vi "Get Array Elements.vi"(6 "Pass non-arrays":bool, 8 "error in (no error)":errorcluster, 10 "Offset":i32, 11 "JSON":string) -> (0 "error out":errorcluster, 1 "<JSON>":string[](array[string]) caption="<JSON>Elements", 2 "Offset past":i32 caption="Offset past Array")   [LabVIEW 2019, in "JSONtext.lvlib"]
doc: "If a JSON Array, returns all elements of the Array.\n\nIf the input JSON is not an Array, this function will return an error, unless \"Pass non-arrays\" is true, in which case the output will be a one-element array containing the input JSON."
uses:
  JSONtext.lvlib
  Parsing/Parsing State.ctl
  Parsing/Advance past Line Ending.vi
  Parsing/Advance past String.vi
  Parsing/Advance past Number.vi
  Parsing/Advance past Array.vi
  Parsing/Advance past Object.vi
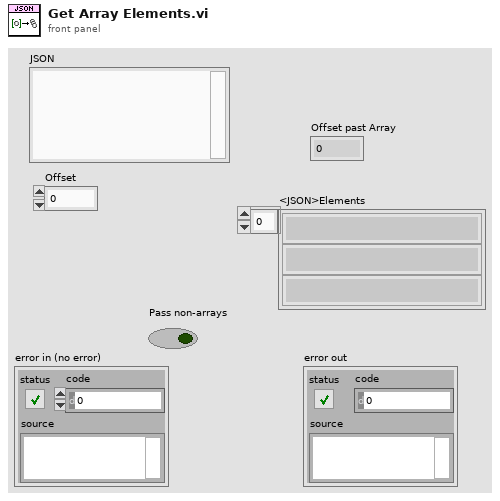
[diagram p1: front panel]
types:
  T1 = typedef "JSONtext.lvlib/Parsing State.ctl" = enum16{"Parser Error", "Object", "Array", "String", "Number/Other", "Leading Whitespace", "Object end", "Array end", "Value end"}
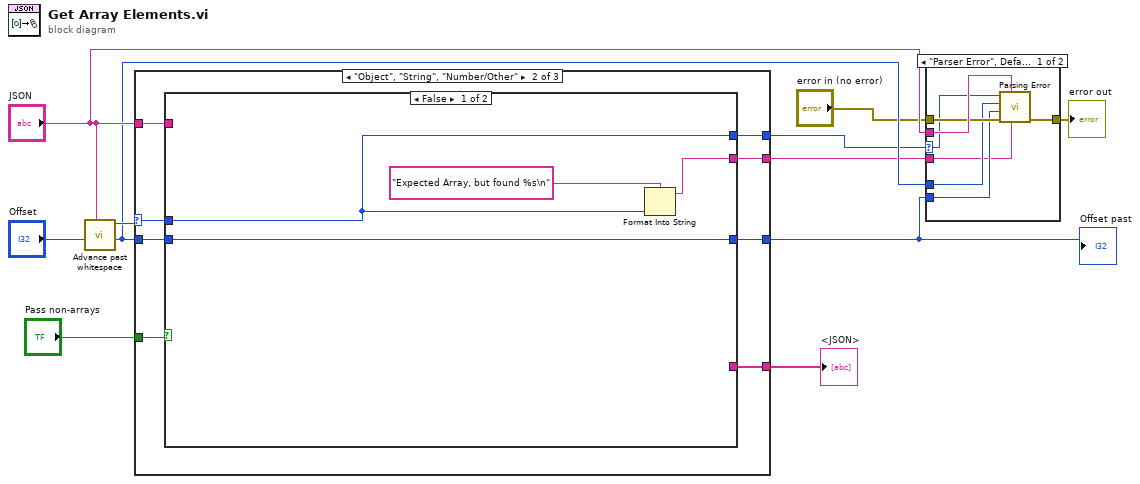
[diagram p0: block diagram]
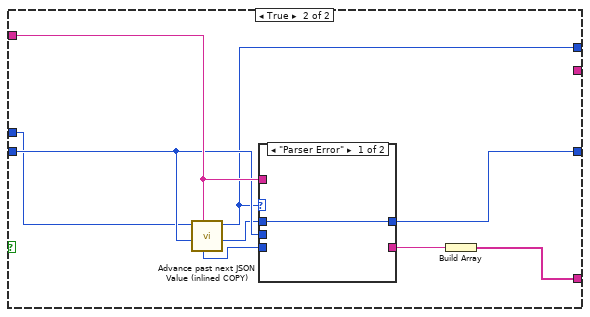
[diagram p4: hidden frame]
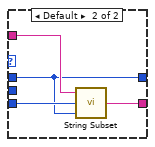
[diagram p5: hidden frame]
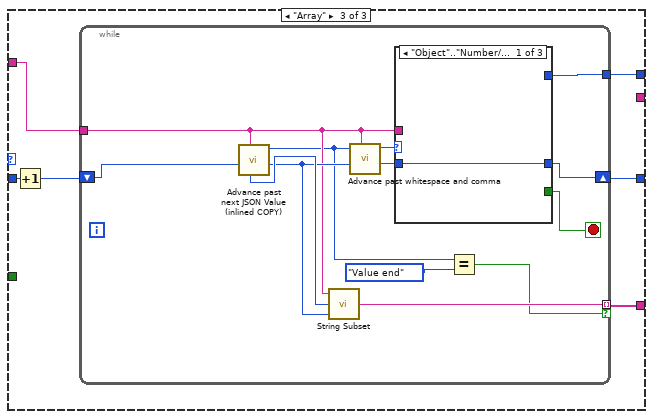
[diagram p6: hidden frame]
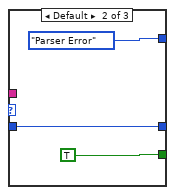
[diagram p7: hidden frame]
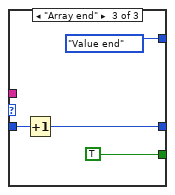
[diagram p8: hidden frame]
diagram:
  n1 = call "Advance past whitespace.vi"("JSON"="JSON", "Offset"="Offset") -> ("Offset of first non-whitespace"=w7:i32, "Parser State"=w9:T1)  [unwired: 7 in, 1 out]
  n2 = case shown="\"Object\", \"String\", \"Number/Other\"" w9 {
    selector: w9 -> [w13 w15 _]
    tunnel: [w13 w17 w45] -> w3
    tunnel: [w12 w18 w44] -> w6
    tunnel: [_ w19 w42] -> w11
    tunnel: "JSON" -> [_ w21 w41]
    tunnel: w7 -> [w12 w20 w40]
    tunnel: "Pass non-arrays" -> [_ w16 _]
    tunnel: [_ w14 _] -> w1
    frame "Parser Error", Default {
    }
    frame "Object", "String", "Number/Other" {
      n3 = case shown="False" w16 {
        tunnel: w21 -> [_ w34]
        tunnel: w20 -> [w25 w33]
        tunnel: [_ w29] -> w19
        tunnel: [w25 w28] -> w18
        tunnel: [w23 w27] -> w17
        tunnel: w15 -> [w23 w26]
        tunnel: [w22 _] -> w14
        frame False {
          n4 = Format Into String(format string="Expected Array, but found %s\n", w23) -> (resulting string=w22:string)  [unwired: 2 in, 1 out]
        }
        frame True {
          n5 = call "Advance past next JSON Value (inlined COPY).vi"("JSON"=w34, "Offset"=w33, "State"=w26) -> ("Offset"=w32:i32, "State"=w27:T1, "Value start"=w31:i32)  [unwired: 4 in, 2 out]
          n6 = case shown="\"Parser Error\"" w27 {
            tunnel: w31 -> [_ w39]
            tunnel: w33 -> [_ _]
            tunnel: w32 -> [w35 w36]
            tunnel: [_ w38] -> w30
            tunnel: w34 -> [_ w37]
            tunnel: [w35 w36] -> w28
            frame "Parser Error" {
            }
            frame Default {
              n7 = call "String Subset.vi"("Offset past End"=w36, "Start offset"=w39, "JSON"=w37) -> ("substring"=w38:string)  [unwired: 2 in]
            }
          }
          n8 = Build Array(w30) -> (w29:string[])
        }
      }
    }
    frame "Array" {
      n9 = Increment(x=w40) -> (x+1=w43:i32)
      n10 = while {
        tunnel: w41 -> [w50]
        shift-right: [w55] -> w44
        shift-left: w43 -> [w56]
        tunnel: [w53] -> w45
        tunnel: [w47] -> w42 mode=indexing if=w46
        stop <- w54 stop-if-true
        n11 = call "Advance past next JSON Value (inlined COPY).vi"("JSON"=w50, "Offset"=w56) -> ("Offset"=w51:i32, "State"=w48:T1, "Value start"=w52:i32)  [unwired: 5 in, 2 out]
        n12 = call "String Subset.vi"("Offset past End"=w51, "Start offset"=w52, "JSON"=w50) -> ("substring"=w47:string)  [unwired: 2 in]
        n13 = call "Advance past whitespace and comma.vi"("JSON"=w50, "Offset"=w51, "State in"=w48) -> ("Offset past match"=w58:i32, "State"=w57:T1)  [unwired: 6 in, 1 out]
        n14 = case shown="\"Object\"..\"Number/Other\"" w57 {
          tunnel: [_ TRUE TRUE] -> w54
          tunnel: [_ Parsing_State."Parser Error" Parsing_State."Value end"] -> w53
          tunnel: w58 -> [w59 w60 w64]
          tunnel: [w59 w60 w63] -> w55
          tunnel: w50 -> [_ _ _]
          frame "Object".."Number/Other" {
          }
          frame Default {
          }
          frame "Array end" {
            n15 = Increment(x=w64) -> (x+1=w63:i32)
          }
        }
        n16 = Equal?(x=w48, y=Parsing_State."Value end") -> (x = y?=w46:bool)
      }
    }
  }
  "Offset past" <- w6
  "<JSON>" <- w11
  n17 = case shown="\"Parser Error\", Default" w3 {
    selector: w3 -> [w68 _]
    tunnel: "JSON" -> [w73 _]
    tunnel: "error in (no error)" -> [w72 w74]
    tunnel: [w71 w74] -> w5
    tunnel: w7 -> [w70 _]
    tunnel: w6 -> [w69 _]
    tunnel: w1 -> [w67 _]
    frame "Parser Error", Default {
      n18 = call "Parsing Error.vi"("initial string"=w67, "JSON"=w73, "error in (no error)"=w72, "Offset past match"=w69, "Value start"=w70, "State"=w68) -> ("error out"=w71:errorcluster)  [unwired: 5 in]
    }
    frame "Value end" {
    }
  }
  "error out" <- w5
